vi "JAS_CameraRead MJPG for Dashboard_2.vi"(6 "Camera Settings":T6={"fps"=30, "compression"=30, "Image Size"=enum."320x240", "Config Shown"=FALSE}, 7 "Camera Settings 2":T3={"Exposure"=enum."Auto", "Exposure (%)"=50.0, "Brightness"=50, "White Balance"=enum."Auto", "Color Temp (K)"=0.0} {"Brightness" min=0 max=100}, 8 "Rec Mode":u16(ring) items=["Stop", "Record", "Playback Panel"], 9 "NT Connection":bool, 10 "Capture Info":T5={"Camera Name"="Camera", "Display Name"="left", {"Save Path"=path "", "Interval (s)"=1.0, "Keep"=180}}, 11 "Image in":T4) -> (1 "perf info":cluster{"Bandwidth (Mbps)":dbl, "fps":dbl}, 2 "Active":bool, 3 "Image\\ out":T4)   [LabVIEW 2025]
doc: "This VI connects to a camera server of the connected robot. It requests images for a given camera name and settings. USB cameras should generally support all settings. IP cameras support only those in Camera Settings cluster. If the settings, name or other settings change, it will close and reopen as needed. The VI should be called repeatedly and it will return with the latest image from the server."
uses:
  <vilib>/vision/Image Controls.llb/IMAQ Image.ctl
  <vilib>/Rock Robotics/WPI/Camera/WPI_CameraExposure Values.ctl
  <vilib>/Rock Robotics/WPI/Camera/WPI_CameraWhite Balance Values.ctl
  <vilib>/Rock Robotics/WPI/Dashboard/WPI_DashboardLogging Global.vi
  JAS_CameraImageSize.ctl
  JAS_CameraSettings Read MJPG.ctl
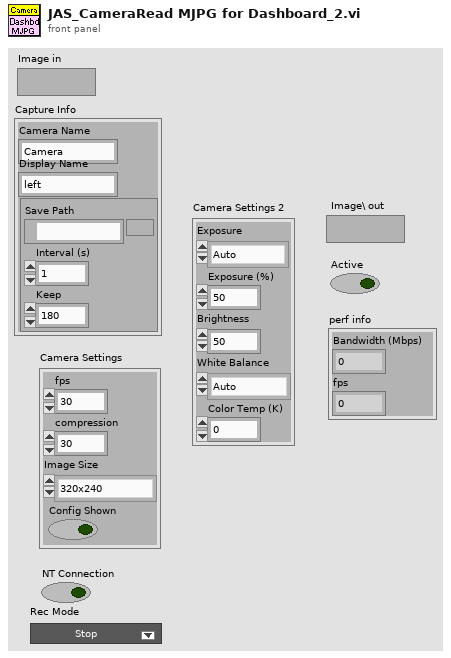
[diagram p1: front panel]
types:
  T1 = typedef "WPI_CameraExposure Values.ctl" = enum16{"Auto", "Flicker-free 50 Hz", "Flicker-free 60 Hz", "Hold current", "Custom"}
  T2 = typedef "WPI_CameraWhite Balance Values.ctl" = enum16{"Auto", "Fixed indoor", "Fixed outdoor 1", "Fixed outdoor 2", "Fixed fluorescent 1", "Fixed fluorescent 2", "Hold current", "Custom"}
  T3 = cluster{"Exposure":T1, "Exposure (%)":dbl, "Brightness":i32, "White Balance":T2, "Color Temp (K)":dbl}
  T4 = typedef "IMAQ Image.ctl" = refnum<image>
  T5 = cluster{"Camera Name":string, "Display Name":string, cluster{"Save Path":path, "Interval (s)":dbl, "Keep":i32}}
  T6 = typedef "JAS_CameraSettings Read MJPG.ctl" = cluster{"fps":i32, "compression":i32, "Image Size":T7, "Config Shown":bool}
  T7 = typedef "JAS_CameraImageSize.ctl" = enum16{"640x480", "640x360", "320x240", "320x180", "160x120", "160x90", "Custom"}
  T8 = cluster{"Save Path":path, "Interval (s)":dbl, "Keep":i32}
  T9 = cluster{"Camera Name":string, "fps":i32, "compression":i32, "Image Size":T7}
  T10 = typedef "IMAQ AVI2 Refnum.ctl" = refnum<k20>
  T11 = cluster{"token string":string, "token string":string}[]
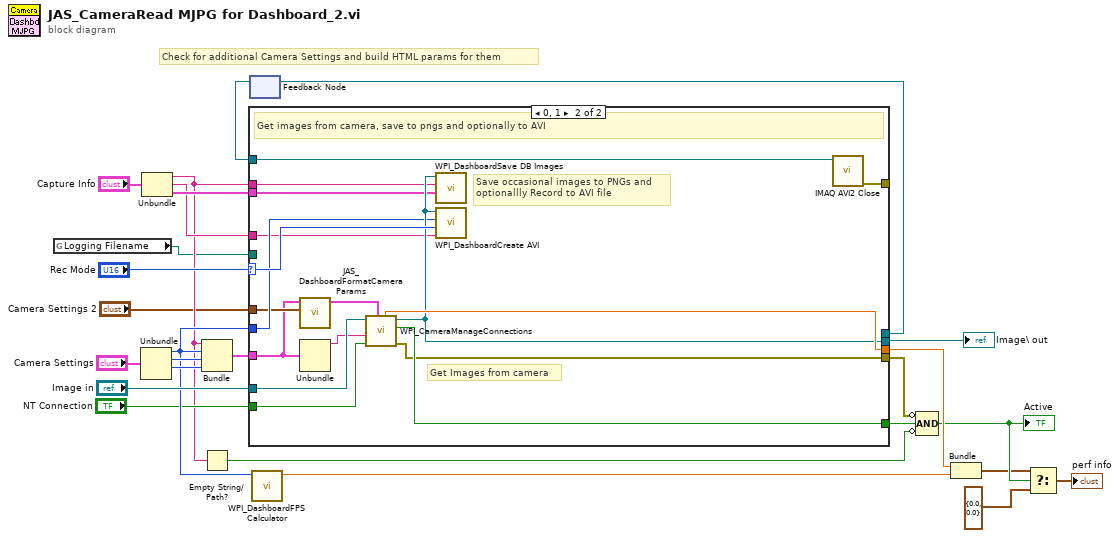
[diagram p0: block diagram]
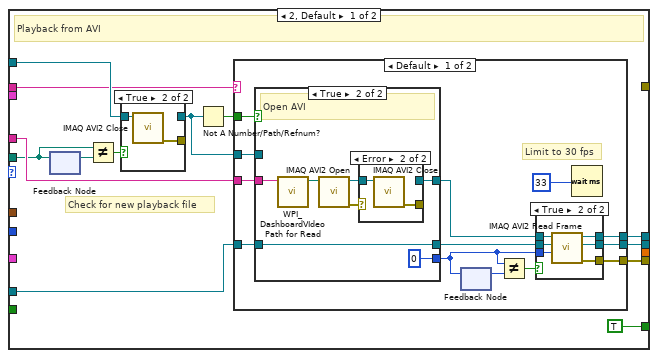
[diagram p2: hidden frame]
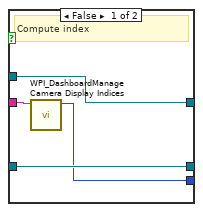
[diagram p5: hidden frame]
diagram:
  # "Check for additional Camera Settings and build HTML params for them"
  n1 = global read "WPI_DashboardLogging Global.vi" "Logging Filename"() -> (w1:path)
  n2 = Unbundle("Camera Settings") -> ("fps"=w18:i32, "compression"=w20:i32, "Image Size"=w19:T7)  [unwired: 1 out]
  n3 = Unbundle("Capture Info") -> ("Camera Name"=w13:string, "Display Name"=w14:string, w15:T8)
  n4 = Bundle("Camera Name"=w13, "fps"=w18, "compression"=w20, "Image Size"=w19) -> (w10:T9)  [unwired: 1 in]
  n5 = Empty String/Path?(string/path=w13) -> (empty?=w8:bool)
  n6 = feedback #1() -> (w23:T10)  [unwired: 1 in]
  n7 = case shown="0, 1" "Rec Mode" {
    selector: "Rec Mode" -> [_ w94]
    tunnel: [_ w96] -> w6
    tunnel: [w39 w91] -> w24
    tunnel: "Image in" -> [w37 w95]
    tunnel: w23 -> [w33 w93]
    tunnel: [w36 _] -> w22
    tunnel: [w35 w89] -> w9
    tunnel: [_ w92] -> _
    tunnel: [TRUE w90] -> w12
    tunnel: w18 -> [_ w88]
    tunnel: "NT Connection" -> [_ w87]
    tunnel: w13 -> [w28 w86]
    tunnel: w15 -> [_ w84]
    tunnel: w14 -> [w29 w85]
    tunnel: "Camera Settings 2" -> [_ w83]
    tunnel: w10 -> [_ w81]
    tunnel: w1 -> [w27 _]
    frame 2, Default {
      # "Check for new playback file"
      # "Playback from AVI"
      n8 = feedback #2() -> (w32:path)  [unwired: 1 in]
      n9 = feedback-in #2(w27) -> ()
      n10 = Not Equal?(x=w27, y=w32) -> (x != y?=w31:bool)
      n11 = case shown="True" w31 {
        tunnel: [w40 _] -> w34
        tunnel: w33 -> [w40 w42]
        tunnel: [_ w41] -> _
        frame False {
        }
        frame True {
          n12 = call "IMAQ AVI2 Close"("AVI Refnum"=w42) -> ("error out"=w41:errorcluster)  [unwired: 10 in]
        }
      }
      n13 = Not A Number/Path/Refnum?(number/path/refnum=w34) -> (NaN/Path/Refnum?=w38:bool)
      n14 = case shown="Default" w28 {
        tunnel: [w55 w78] -> w39
        tunnel: w38 -> [w54 _]
        tunnel: w37 -> [w51 w78]
        tunnel: [w50 w79] -> w36
        tunnel: [w49 _] -> w35
        tunnel: w29 -> [w48 _]
        tunnel: w34 -> [w47 w79]
        frame Default {
          # "Limit to 30 fps"
          n15 = case shown="True" w54 {
            tunnel: [w67 w72] -> w53
            tunnel: w47 -> [w67 _]
            tunnel: [w66 w74] -> w52
            tunnel: w51 -> [w66 w74]
            tunnel: [w64 0 ("Video Frame #")] -> w44
            tunnel: w48 -> [w65 w69]
            frame False {
              # "Compute index"
              n16 = call <vilib>:"WPI_DashboardManage Camera Display Indices.vi"("Display Name"=w65) -> ("index of element"=w64:i32)  [unwired: 10 in]
            }
            frame True {
              # "Open AVI"
              n17 = call <vilib>:"WPI_DashboardVIdeo Path for Read.vi"("Display Name"=w69) -> ("Video Path"=w68:path)  [unwired: 10 in]
              n18 = call "IMAQ AVI2 Open"("AVI File Path"=w68) -> ("error out"=w73:errorcluster, "AVI Refnum"=w71:T10)  [unwired: 9 in]
              n19 = case shown="Error" w73 {
                tunnel: [w75 _] -> w72
                tunnel: w71 -> [w75 w77]
                tunnel: [_ w76] -> _
                frame No Error {
                }
                frame Error {
                  n20 = call "IMAQ AVI2 Close"("AVI Refnum"=w77) -> ("error out"=w76:errorcluster)  [unwired: 10 in]
                }
              }
            }
          }
          n21 = feedback #3() -> (w45:i32)  [unwired: 1 in]
          n22 = feedback-in #3(w44) -> ()
          n23 = Not Equal?(x=w44, y=w45) -> (x != y?=w46:bool)
          n24 = case shown="True" w46 {
            tunnel: [w56 w63] -> w55
            tunnel: w53 -> [w57 w62]
            tunnel: w52 -> [w56 w61]
            tunnel: [w57 w60] -> w50
            tunnel: [_ w59] -> w49
            tunnel: w44 -> [_ w58]
            frame False {
            }
            frame True {
              n25 = call "IMAQ AVI2 Read Frame"("Frame Number"=w58, "Image"=w61, "AVI Refnum"=w62) -> ("error out"=w59:errorcluster, "Image Out"=w63:T4, "AVI Refnum (duplicate)"=w60:T10)  [unwired: 6 in]
            }
          }
          n26 = Wait (ms)(milliseconds to wait=33) -> ()  [unwired: 1 out]
        }
        frame "" {
          # "No file name to playback"
        }
      }
    }
    frame 0, 1 {
      # "Get Images from camera"
      # "Save occasional images to PNGs and\noptionallly Record to AVI file"
      # "Get images from camera, save to pngs and optionally to AVI"
      n27 = call "JAS_DashboardFormatCameraParams.vi"("Camera Settings 2"=w83, "Camera Settings"=w81) -> ("parameter pairs"=w82:T11)  [unwired: 9 in]
      n28 = Unbundle(w81) -> ("Camera Name"=w80:string)  [unwired: 3 out]
      n29 = call <vilib>:"WPI_CameraManageConnections.vi"("parameters"=w82, "NT Connection"=w87, "Camera Name"=w80, "Image in"=w95) -> ("error out"=w89:errorcluster, "Active"=w90:bool, "Image out"=w91:T4, "Bandwidth (Mbps)"=w96:dbl)  [unwired: 4 in]
      n30 = call <vilib>:"WPI_DashboardSave DB Images.vi"("Save Info"=w84, "Camera Name"=w86, "Image"=w91) -> ()  [unwired: 7 in]
      n31 = call <vilib>:"WPI_DashboardCreate AVI.vi"("Display Name"=w85, "Recording"=w94, "frames per second"=w88, "Image"=w91) -> ()  [unwired: 8 in]
      n32 = call "IMAQ AVI2 Close"("AVI Refnum"=w93) -> ("error out"=w92:errorcluster)  [unwired: 10 in]
    }
  }
  "Image\\ out" <- w24
  n33 = feedback-in #1(w22) -> ()
  n34 = call <vilib>:"WPI_DashboardFPS Calculator.vi"("Average Count"=w18) -> ("fps"=w7:dbl)  [unwired: 9 in, 1 out]
  n35 = Compound Arithmetic op=AND(invert w9, w12, invert w8) -> (w5:bool)
  "Active" <- w5
  n36 = Bundle("Bandwidth (Mbps)"=w6, "fps"=w7) -> (w3:cluster{"Bandwidth (Mbps)":dbl, "fps":dbl})  [unwired: 1 in]
  n37 = Select(t=w3, s=w5, f=cluster{"Bandwidth (Mbps)":dbl, "fps":dbl} {"Bandwidth (Mbps)"=0.0, "fps"=0.0}) -> (s? t:f=→"perf info":cluster{"Bandwidth (Mbps)":dbl, "fps":dbl})
